vi "2283_Outputs autonomo.vi"() -> ()   [LabVIEW 2014]
panel:
  in  "Outputs autonomo":T1
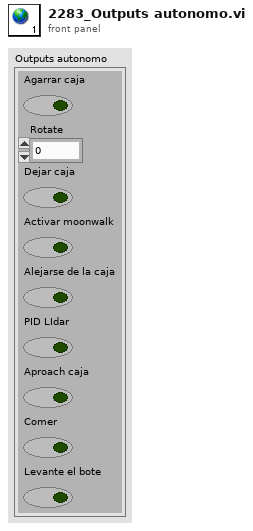
[diagram p1: front panel]
types:
  T1 = cluster{"Agarrar caja":bool, "Rotate":dbl, "Dejar caja":bool, "Activar moonwalk":bool, "Alejarse de la caja":bool, "PID LIdar":bool, "Aproach caja":bool, "Comer":bool, "Levante el bote":bool}
diagram:
